vi "RetrieveJobAndMachineOrders.vi"(8 "error in (no error)":errorcluster, 9 "Number of Machines":i32, 10 "Schedule":u16[](array[numeric]), 11 "OSSP_Problem in":refnum<class "OSSP_Problem.lvclass">) -> (0 "error out":errorcluster, 2 "Mo4J":u16[][](array[numeric]), 3 "JO4M":u16[][](array[numeric]))   [LabVIEW 2013, in "GA.lvclass"]
uses:
  GA.lvclass
  OSSP_Problem.lvclass
  OSSP_Problem.lvclass/OSSP_Problem.ctl
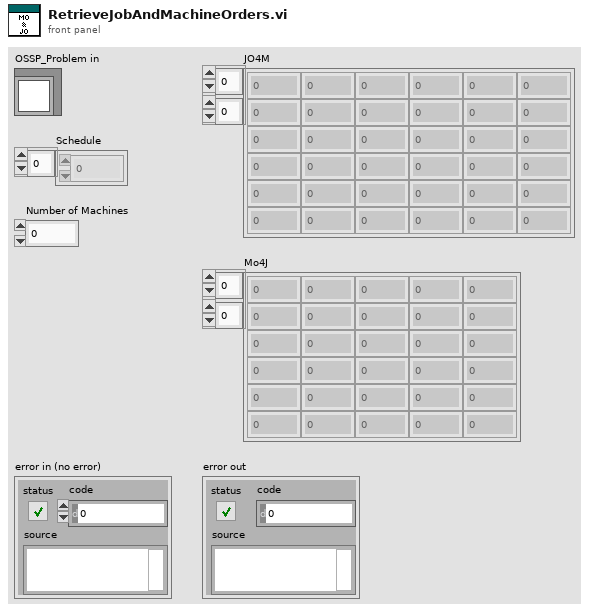
[diagram p1: front panel]
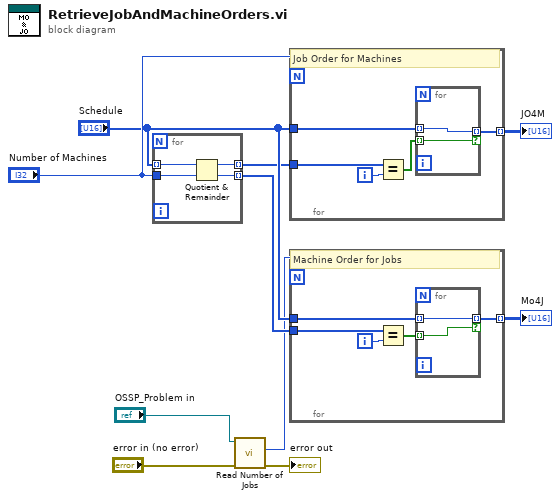
[diagram p0: block diagram]
diagram:
  n1 = for {
    tunnel: "Schedule" -> [w14] mode=indexing
    tunnel: "Number of Machines" -> [w13]
    tunnel: [w12] -> w5 mode=indexing
    tunnel: [w11] -> w3 mode=indexing
    n2 = Quotient & Remainder(x=w14, y=w13) -> (x-y*floor(x/y)=w12:i32, floor(x/y)=w11:i32)
  }
  n3 = call "Read Number of Jobs.vi"("error in (no error)"="error in (no error)", "OSSP_Problem in"="OSSP_Problem in") -> ("error out"=→"error out":errorcluster, "Number of Jobs"=w1:i32)  [unwired: 7 in, 1 out]
  n4 = for {
    N: "Number of Machines" -> [_]
    tunnel: "Schedule" -> [w16]
    tunnel: w5 -> [w19]
    tunnel: [w15] -> w4 mode=indexing
    i -> [w18]
    # "Job Order for Machines"
    n5 = Equal?(x=w19, y=w18) -> (x = y?=w17:bool[])
    n6 = for {
      tunnel: w17 -> [w20] mode=indexing
      tunnel: w16 -> [w21] mode=indexing
      tunnel: [w21] -> w15 mode=indexing if=w20
    }
  }
  "JO4M" <- w4
  n7 = for {
    N: w1 -> [_]
    tunnel: "Schedule" -> [w23]
    tunnel: w3 -> [w26]
    tunnel: [w22] -> w2 mode=indexing
    i -> [w25]
    # "Machine Order for Jobs"
    n8 = Equal?(x=w26, y=w25) -> (x = y?=w24:bool[])
    n9 = for {
      tunnel: w24 -> [w27] mode=indexing
      tunnel: w23 -> [w28] mode=indexing
      tunnel: [w28] -> w22 mode=indexing if=w27
    }
  }
  "Mo4J" <- w2
